vi "Main VI 2.vi"() -> ()   [LabVIEW 2016]
panel:
  in  "stop":bool
  # "Main VI 2"
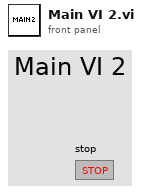
[diagram p1: front panel]
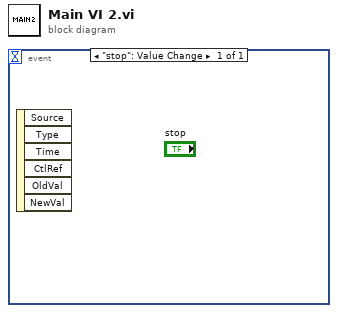
[diagram p0: block diagram]
diagram:
  n1 = event shown="[0] \"stop\": Value Change" {
    selector: _ -> [_]
    dyn-events: _ -> [_]
    timeout: _ -> [_]
    event "stop": Value Change {
      n2 = event-data() -> ()  [unwired: 1 in, 6 out]
    }
  }
